vi "hamamatsuRun.vi"() -> ()   [LabVIEW 2017]
uses:
  globalDevices.vi
  globalUtilities.vi
  <userlib>/Hamamatsu Video Capture/tm_waitnextframe_40.vi
  <userlib>/Hamamatsu Video Capture/tm_getframe16_40.vi
  <vilib>/Analysis/baseanly.llb/Std Deviation and Variance.vi
  <userlib>/Hamamatsu Video Capture/tm_stopcapture_40.vi
panel:
  out "frameCount":i32[](array[numeric])
  out "XY Graph":cluster{"Array of Double":dbl[], dbl[]}(graph)
  in  "stop 2":bool
  out "Waveform Graph":dbl[](graph)
  in  "stop":bool
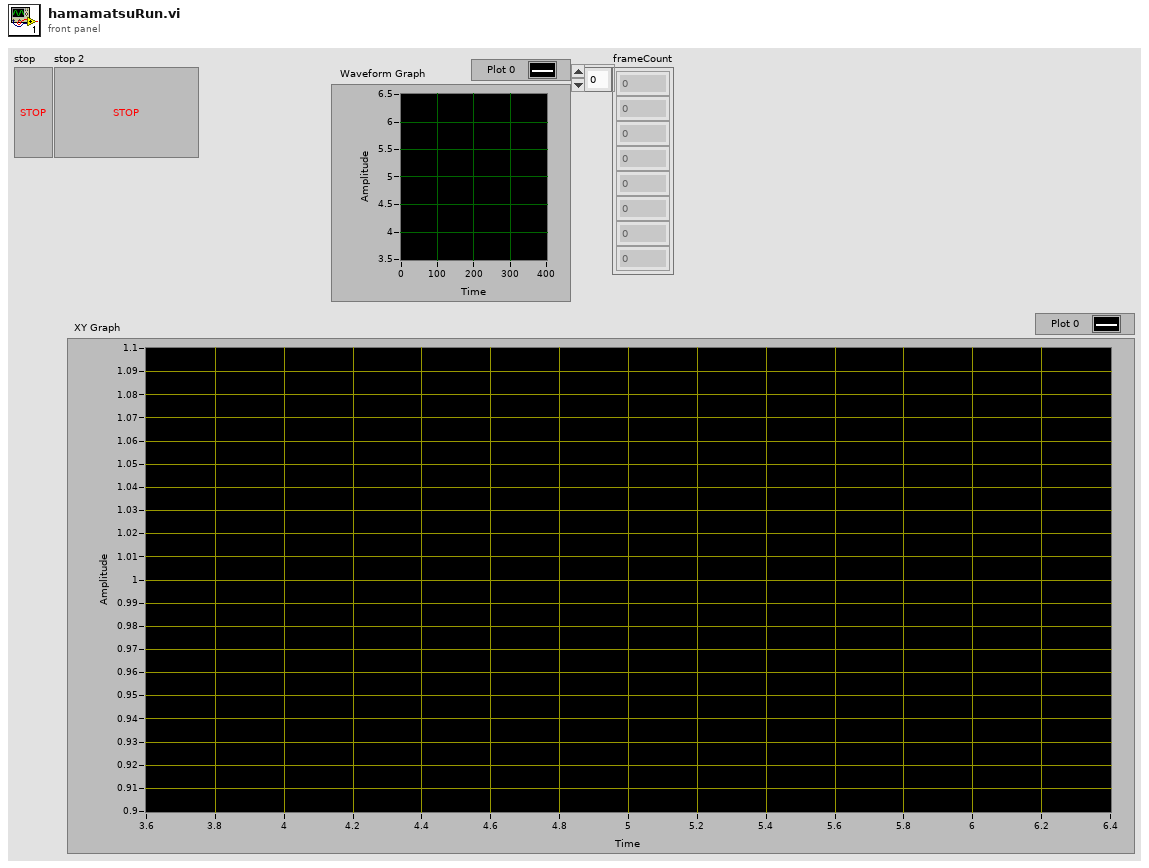
[diagram p1: front panel]
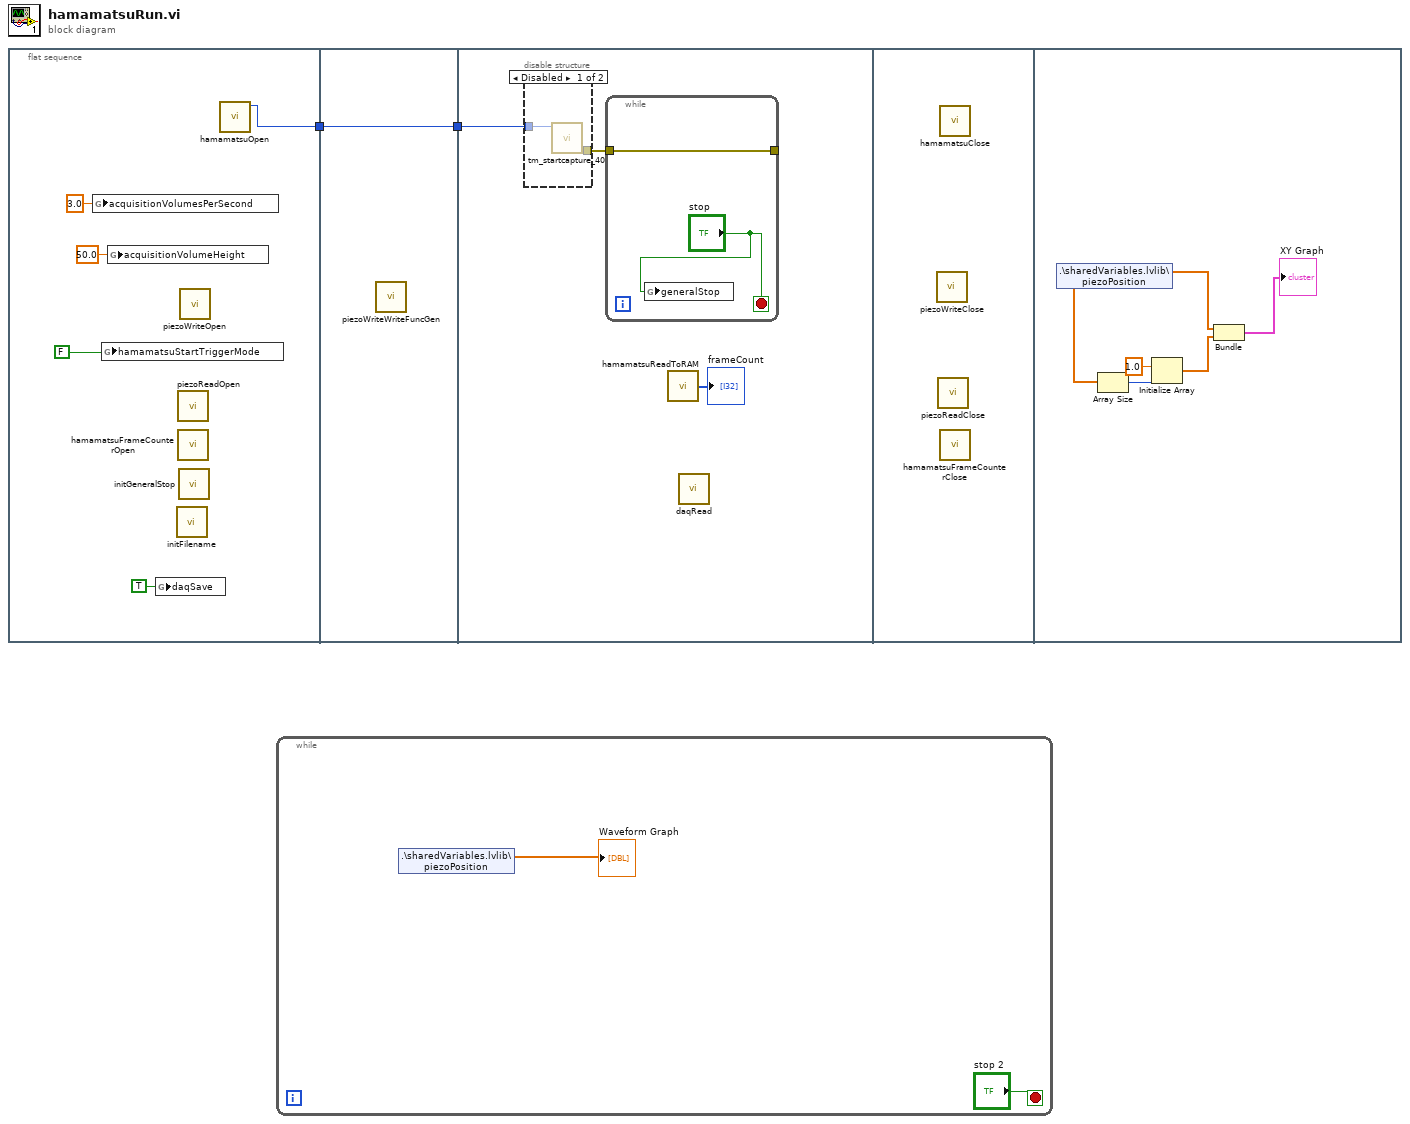
[diagram p0: block diagram]
diagram:
  n1 = flat-sequence {
    tunnel: [w6] -> w2
    tunnel: w2 -> [w8]
    tunnel: [w8] -> w1
    tunnel: w1 -> [w10]
    frame #0 {
      n2 = global write "globalUtilities.vi" "acquisitionVolumesPerSecond"(3.0 ("acquisitionVolumesPerSecond")) -> ()
      n3 = global write "globalDevices.vi" "hamamatsuStartTriggerMode"(FALSE ("hamamatsuStartTriggerMode")) -> ()
      n4 = global write "globalUtilities.vi" "acquisitionVolumeHeight"(50.0 ("acquisitionVolumeHeight")) -> ()
      n5 = global write "globalUtilities.vi" "daqSave"(TRUE ("daqSave")) -> ()
      n6 = call "initFilename.vi"() -> ()  [unwired: 2 in, 1 out]
      n7 = call "piezoReadOpen.vi"() -> ()  [unwired: 6 in]
      n8 = call "hamamatsuFrameCounterOpen.vi"() -> ()  [unwired: 12 in]
      n9 = call "initGeneralStop.vi"() -> ()  [unwired: 1 in]
      n10 = call "piezoWriteOpen.vi"() -> ()  [unwired: 2 in]
      n11 = call "hamamatsuOpen.vi"() -> ("Handle out"=w6:u32)  [unwired: 3 out]
    }
    frame #1 {
      n12 = call "piezoWriteWriteFuncGen.vi"() -> ()  [unwired: 12 in]
    }
    frame #2 {
      n13 = disable-structure shown="Disabled" {
        disable-tunnel: [w13 _] -> w11
        disable-tunnel: w10 -> [w12 _]
        frame Disabled {
          n14 = call <userlib>:"tm_startcapture_40.vi"("Handle in"=w12) -> ("error out"=w13:errorcluster)  [unwired: 9 in, 1 out]
        }
        frame Enabled {
        }
      }
      n15 = while {
        tunnel: w11 -> [w15]
        tunnel: [w15] -> _
        stop <- "stop" stop-if-true
        n16 = global write "globalUtilities.vi" "generalStop"("stop") -> ()
      }
      n17 = call "hamamatsuReadToRAM.vi"() -> ("frameCount"=→"frameCount":i32[])  [unwired: 1 in, 2 out]
      n18 = call "daqRead.vi"() -> ()  [unwired: 3 in]
    }
    frame #3 {
      n19 = call "piezoWriteClose.vi"() -> ()  [unwired: 1 in]
      n20 = call "piezoReadClose.vi"() -> ()  [unwired: 1 in]
      n21 = call "hamamatsuClose.vi"() -> ()  [unwired: 1 out]
      n22 = call "hamamatsuFrameCounterClose.vi"() -> ()  [unwired: 12 in]
    }
    frame #4 {
      n23 = shared-variable ".\\sharedVariables.lvlib\\piezoPosition"() -> (w18:dbl[])  [unwired: 1 in, 1 out]
      n24 = Array Size(array=w18) -> (size(s)=w20:i32)
      n25 = Initialize Array(1.0 ("element"), w20) -> (w17:dbl[])
      n26 = Bundle("Array of Double"=w18, w17) -> (→"XY Graph":cluster{"Array of Double":dbl[], dbl[]})  [unwired: 1 in]
    }
  }
  n27 = while {
    stop <- "stop 2" stop-if-true
    n28 = shared-variable ".\\sharedVariables.lvlib\\piezoPosition"() -> (→"Waveform Graph":dbl[])  [unwired: 1 in, 1 out]
  }
